vi "Create Thread Parameters.vi"(8 "error in (no error)":errorcluster, 9 "id":i32, 10 "processor":i32=-2, 11 "priority":i32=100) -> (0 "error out":errorcluster, 3 "Thread Parameters":refnum<class "Thread Parameters.lvclass">)   [LabVIEW 2017, in "DSF Core.lvlib" / "Thread Parameters.lvclass"]
uses:
  Thread Parameters.lvclass
  Thread Parameters.lvclass/Thread Parameters.ctl
  Invalid ID.vi
  Invalid Priority.vi
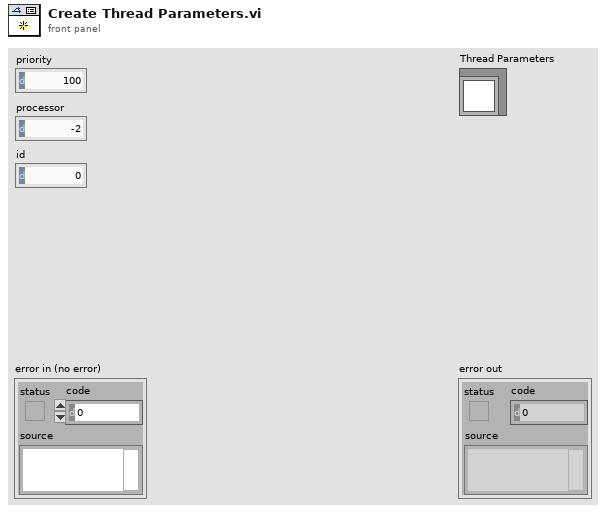
[diagram p1: front panel]
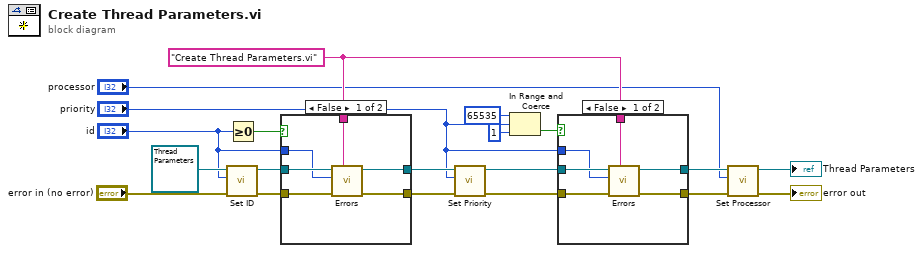
[diagram p0: block diagram]
diagram:
  w7 = "Create Thread Parameters.vi" ("error source vi name")
  n1 = call "Set ID.vi"("id"="id", "Plugin in"=refnum<class "Thread Parameters.lvclass"> refnum ("Thread Parameters in")) -> ("Plugin out"=w15:refnum<class "Thread Parameters.lvclass">)  [unwired: 9 in]
  n2 = Greater Or Equal To 0?(x="id") -> (x >= 0?=w12:bool)
  n3 = case shown="False" w12 {
    tunnel: w15 -> [w23 w25]
    tunnel: [w22 w25] -> w14
    tunnel: [w21 w24] -> w8
    tunnel: "error in (no error)" -> [w20 w24]
    tunnel: w7 -> [w19 _]
    tunnel: "id" -> [w18 _]
    frame False {
      n4 = call-poly "Errors.vi"("error source vi name"=w19, "error in (no error)"=w20, "id"=w18, "Thread Parameters in"=w23) -> ("error out"=w21:errorcluster, "Thread Parameters out"=w22:refnum<class "Thread Parameters.lvclass">)  [unwired: 6 in]
    }
    frame True {
    }
  }
  n5 = call "Set Priority.vi"("Priority"="priority", "Thread Parameters in"=w14) -> ("Thread Parameters out"=w10:refnum<class "Thread Parameters.lvclass">)  [unwired: 9 in]
  n6 = In Range and Coerce(upper limit=65535, x="priority", lower limit=1) -> (In Range?=w2:bool)  [unwired: 1 out]
  n7 = case shown="False" w2 {
    tunnel: w10 -> [w31 w33]
    tunnel: [w30 w33] -> w9
    tunnel: [w29 w32] -> w1
    tunnel: w8 -> [w28 w32]
    tunnel: w7 -> [w27 _]
    tunnel: "priority" -> [w26 _]
    frame False {
      n8 = call-poly "Errors.vi"("error source vi name"=w27, "error in (no error)"=w28, "priority"=w26, "Thread Parameters in"=w31) -> ("error out"=w29:errorcluster, "Thread Parameters out"=w30:refnum<class "Thread Parameters.lvclass">)  [unwired: 6 in]
    }
    frame True {
    }
  }
  "error out" <- w1
  n9 = call "Set Processor.vi"("Processor"="processor", "Thread Parameters in"=w9) -> ("Thread Parameters out"=→"Thread Parameters":refnum<class "Thread Parameters.lvclass">)  [unwired: 9 in]
